vi "Leitura Weather160.vi"() -> (0 "Erro de Leitura=True":bool, 2 "Array":string[](array[string]))   [LabVIEW 2018]
uses:
  Global_Telescopio.vi
  <vilib>/Utility/error.llb/whitespace.ctl
  Shared_160.lvlib
panel:
  out "sizeFile":i32
  out "sizeCte":i32
  out "error out":errorcluster
  out "Ultima linha":string
  out "Saida":string
  # "Temp     Hi      Low     Out    Dew  Wind  Wind   Wind    Hi    Hi   Wind   Heat  THW  THSW             Solar   Solar   Hi Solar   UV    UV      Hi     Heat    Cool    In           In          In       In    Wind  Wind   ISS   Arc.\n  Date    Time     Out   Temp   Temp   Hum    Pt.  Speed   Dir      Run  Speed   Dir  Chill  Index  Index  Index    Bar     Rad.  Energy    Rad.  Index  Dose   UV     D-D     D-D    Temp   Hum    Dew   Heat     ET   Samp   Tx   Recept  Int."
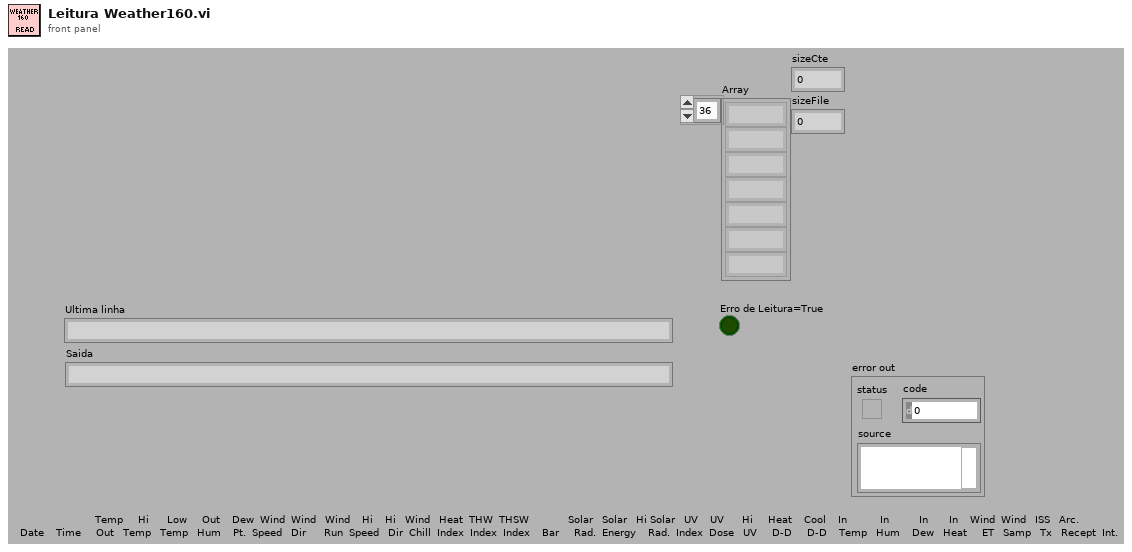
[diagram p1: front panel]
types:
  T1 = enum16{"open", "open or create", "create or replace", "create"}
  T2 = cluster{"broker":string, "version":string, "date":string, "hour":string, "outTemp":string, "hiTemp":string, "lowTemp":string, "outHumidity":string, "dewOut":string, "windSpeed":string, "windDirection":string, "windRun":string, "hiSpeed":string, "hiDir":string, "windChill":string, "heatIndex":string, "THWIndex":string, "THSIndex":string, "pressure":string, "rain":string, "rainRate":string, "solarRad":string, "solarEnergy":string, "hiSolarRad":string, "UVIndex":string, "UVDose":string, "hiUV":string, "headDD":string, "coolDD":string, "inTemp":string, "inHumidity":string, "inHeat":string, "inEMC":string, "inAirDensity":string, "2ndTemp":string, "2ndHumidity":string, "ET":string, "leaf":string, "windSamp":string, "windTx":string, "ISSRecept":string, "dewIn":string, "arcInt":string}
  T3 = typedef "whitespace.ctl" = u16
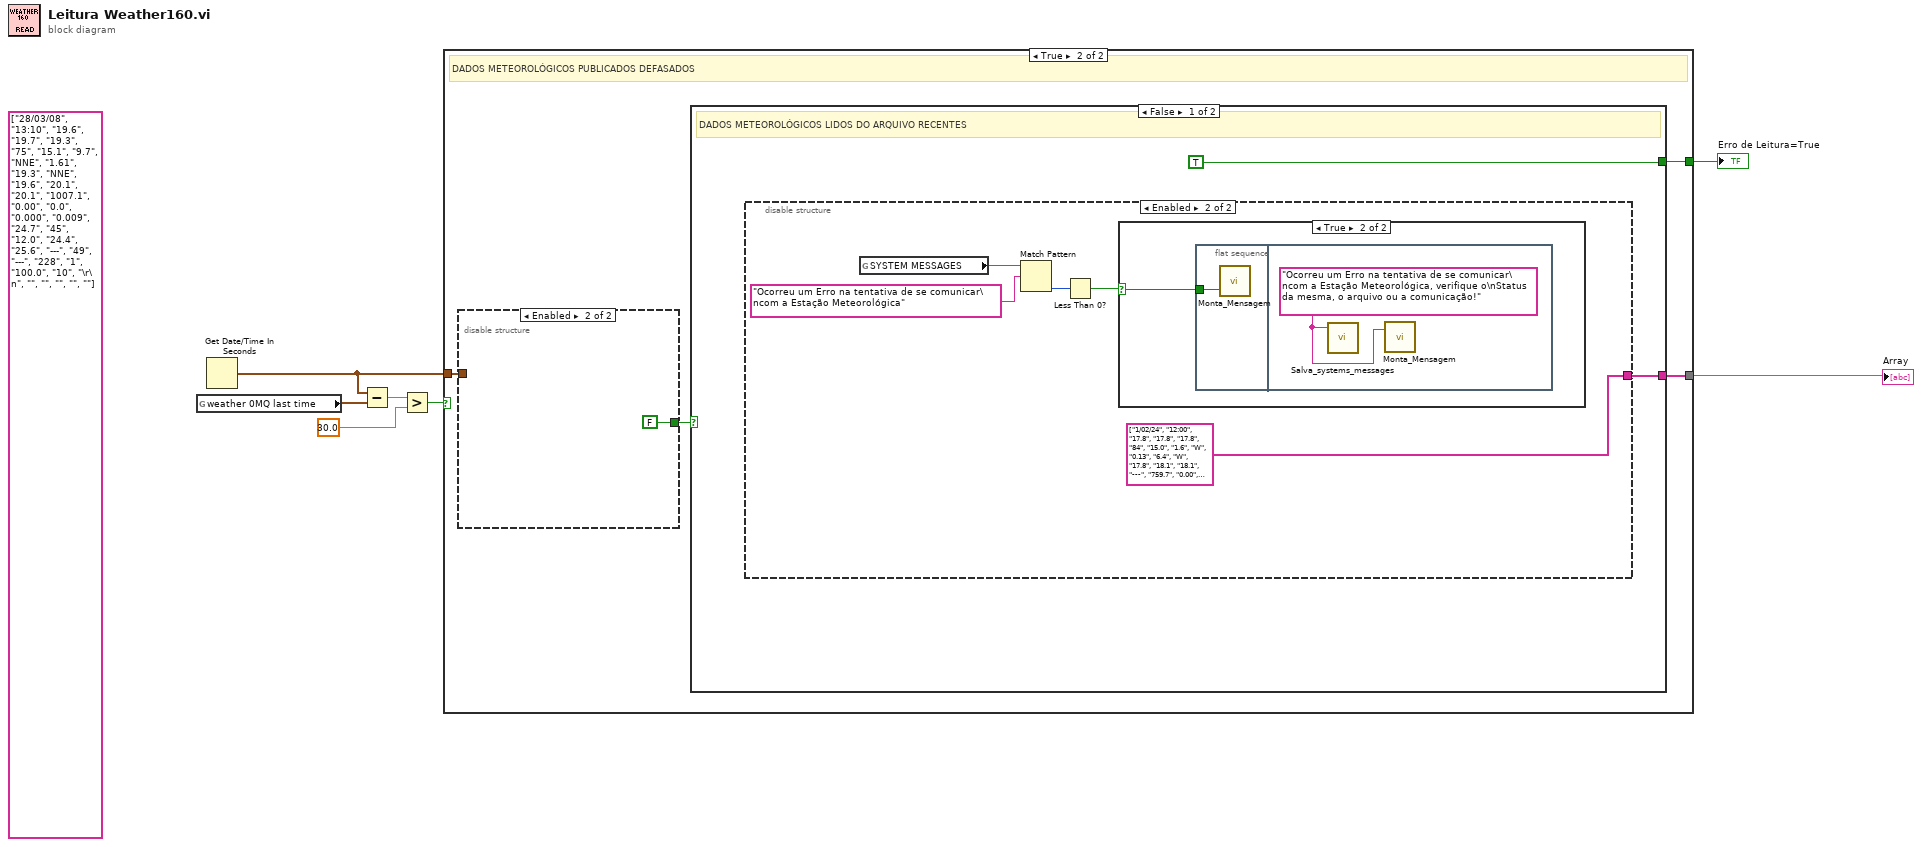
[diagram p0: block diagram]
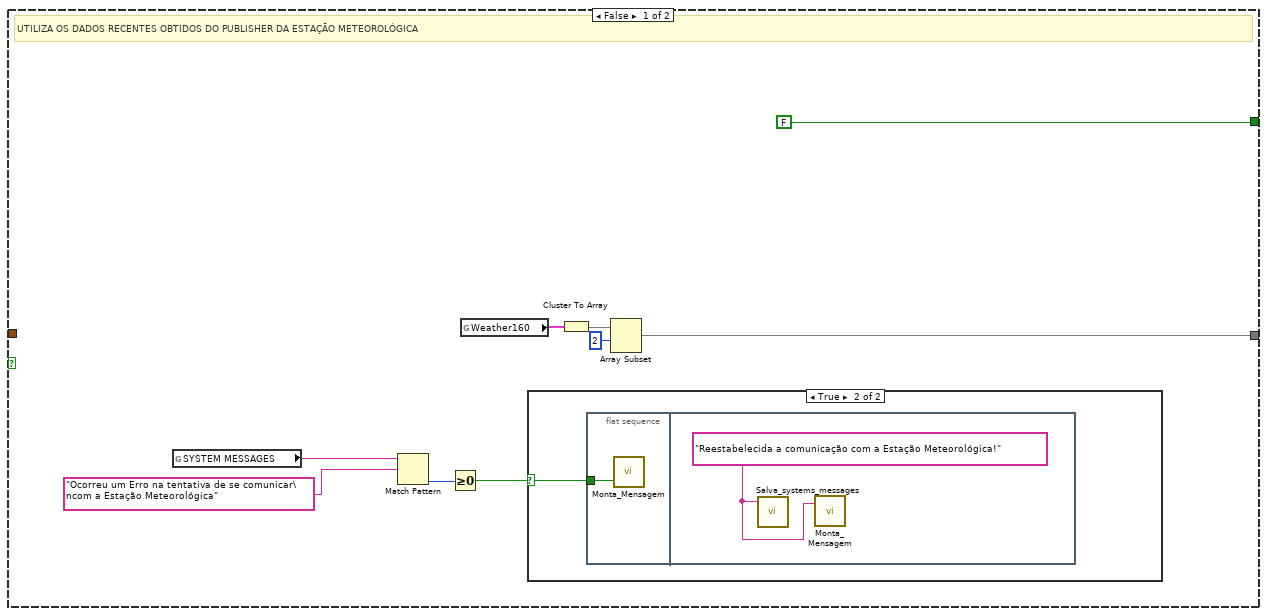
[diagram p2: hidden frame]
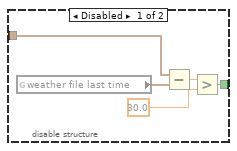
[diagram p4: hidden frame]
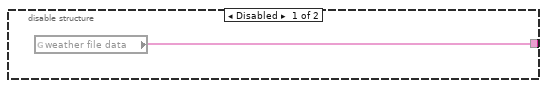
[diagram p5: hidden frame]
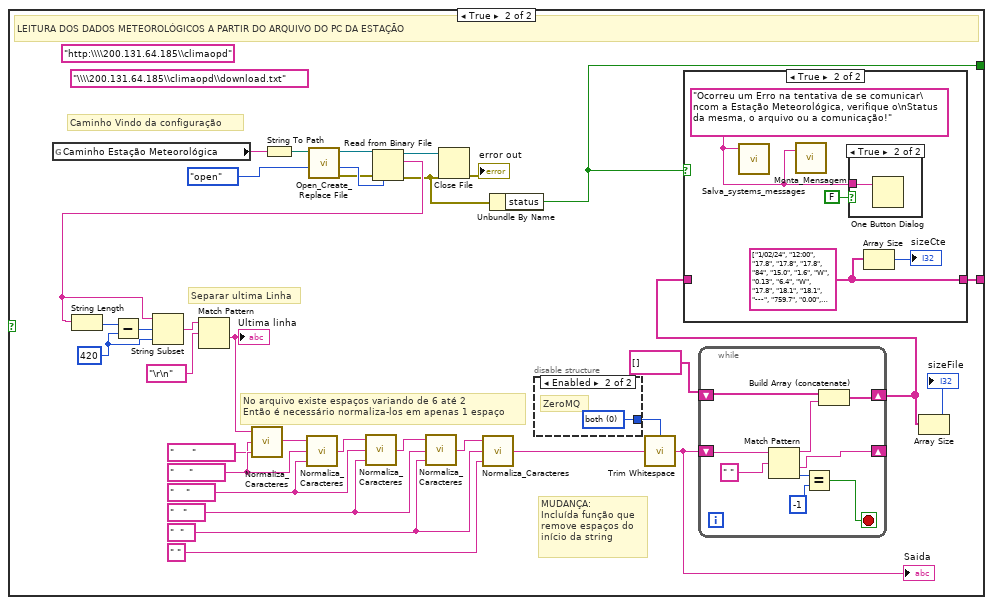
[diagram p7: hidden frame]
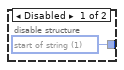
[diagram p8: hidden frame]
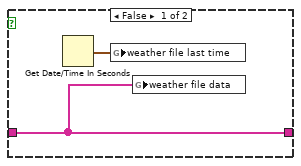
[diagram p9: hidden frame]
diagram:
  (unwired) string[] ["28/03/08", "13:10", "19.6", "19.7", "19.3", "75", "15.1", "9.7", "NNE", "1.61", "19.3", "NNE", "19.6", "20.1", "20.1", "1007.1", "0.00", "0.0", "0.000", "0.009", "24.7", "45", "12.0", "24.4", "25.6", "---", "49", "---", "228", "1", "100.0", "10", "\r\n", "", "", "", "", ""] ("Array 2")
  n1 = global read "Global_Telescopio.vi" "weather 0MQ last time"() -> (w6:timestamp)
  n2 = Get Date/Time In Seconds() -> (seconds since 1Jan1904=w3:timestamp)
  n3 = Subtract(x=w3, y=w6) -> (x-y=w5:dbl)
  n4 = Greater?(x=w5, y=30.0) -> (0:w1:bool)
  n5 = case shown="True" w1 {
    tunnel: [w13 w23] -> w7
    tunnel: w3 -> [_ w22]
    tunnel: [FALSE w20] -> w2
    frame False {
      # "UTILIZA OS DADOS RECENTES OBTIDOS DO PUBLISHER DA ESTAÇÃO METEOROLÓGICA"
      n6 = global read "Global_Telescopio.vi" "SYSTEM MESSAGES"() -> (w11:string)
      n7 = Match Pattern(string=w11, regular expression="Ocorreu um Erro na tentativa de se comunicar\ncom a Estação Meteorológica" ("message")) -> (offset past match=w12:i32)  [unwired: 1 in, 3 out]
      n8 = Greater Or Equal To 0?(x=w12) -> (x >= 0?=w9:bool)
      n9 = global read "Global_Telescopio.vi" "Weather160"() -> (w16:T2)
      n10 = case shown="True" w9 {
        selector: w9 -> [_ w17]
        frame False {
        }
        frame True {
          n11 = flat-sequence {
            tunnel: w17 -> [w18]
            frame #0 {
              n12 = call "Monta_Mensagem.vi"("Zerar"=w18) -> ()  [unwired: 2 in]
            }
            frame #1 {
              w19 = "Reestabelecida a comunicação com a Estação Meteorológica!" ("message")
              n13 = call "Salva_systems_messages.vi"("Mensagem"=w19) -> ()  [unwired: 5 in]
              n14 = call "Monta_Mensagem.vi"("Mensagem"=w19) -> ()  [unwired: 2 in]
            }
          }
        }
      }
      n15 = Cluster To Array(cluster=w16) -> (array=w15:string[])
      n16 = Array Subset(array=w15, index=2) -> (w13:string[])  [unwired: 1 in]
    }
    frame True {
      # "DADOS METEOROLÓGICOS PUBLICADOS DEFASADOS"
      n17 = disable-structure shown="Enabled" {
        disable-tunnel: w22 -> [w27 _]
        disable-tunnel: [w24 FALSE] -> w21
        frame Disabled {
          n18 = global read "Global_Telescopio.vi" "weather file last time"() -> (w26:timestamp)
          n19 = Subtract(x=w27, y=w26) -> (x-y=w28:dbl)
          n20 = Greater?(x=w28, y=30.0) -> (0:w24:bool)
        }
        frame Enabled {
        }
      }
      n21 = case shown="False" w21 {
        tunnel: [w31 w47] -> w23
        tunnel: [TRUE w42] -> w20
        frame False {
          # "DADOS METEOROLÓGICOS LIDOS DO ARQUIVO RECENTES"
          n22 = disable-structure shown="Enabled" {
            disable-tunnel: [w32 string[] ["1/02/24", "12:00", "17.8", "17.8", "17.8", "84", "15.0", "1.6", "W", "0.13", "6.4", "W", "17.8", "18.1", "18.1", "---", "759.7", "0.00", "0.0", "302", "2.16", "364", "3.2", "0.11", "3.6", "0.002", "0.000", "22.6", "64", "15.5", "22.8", "11.65", "1.1730", "21.7", "58", "0.15", "0", "114", "1", "100.0", "5"] ("Array 2")] -> w31
            frame Disabled {
              n23 = global read "Global_Telescopio.vi" "weather file data"() -> (w32:string[])
            }
            frame Enabled {
              n24 = global read "Global_Telescopio.vi" "SYSTEM MESSAGES"() -> (w36:string)
              n25 = Match Pattern(string=w36, regular expression="Ocorreu um Erro na tentativa de se comunicar\ncom a Estação Meteorológica" ("message")) -> (offset past match=w33:i32)  [unwired: 1 in, 3 out]
              n26 = Less Than 0?(x=w33) -> (x < 0?=w34:bool)
              n27 = case shown="True" w34 {
                selector: w34 -> [_ w38]
                frame False {
                }
                frame True {
                  n28 = flat-sequence {
                    tunnel: w38 -> [w39]
                    frame #0 {
                      n29 = call "Monta_Mensagem.vi"("Zerar"=w39) -> ()  [unwired: 2 in]
                    }
                    frame #1 {
                      w40 = "Ocorreu um Erro na tentativa de se comunicar\ncom a Estação Meteorológica, verifique o\nStatus da mesma, o arquivo ou a comunicação!" ("message")
                      n30 = call "Salva_systems_messages.vi"("Mensagem"=w40) -> ()  [unwired: 5 in]
                      n31 = call "Monta_Mensagem.vi"("Mensagem"=w40) -> ()  [unwired: 2 in]
                    }
                  }
                }
              }
            }
          }
        }
        frame True {
          w56 = 420 ("y")
          (unwired) "http:\\\\200.131.64.185\\climaopd"
          (unwired) "\\\\200.131.64.185\\climaopd\\download.txt" ("caminho final")
          w63 = "     "
          w67 = "  "
          w64 = "    "
          w68 = "   "
          # "MUDANÇA:\nIncluída função que\nremove espaços do\ninício da string"
          # "Caminho Vindo da configuração"
          # "Separar ultima Linha"
          # "No arquivo existe espaços variando de 6 até 2\nEntão é necessário normaliza-los em apenas 1 espaço"
          # "LEITURA DOS DADOS METEOROLÓGICOS A PARTIR DO ARQUIVO DO PC DA ESTAÇÃO"
          n32 = global read "Global_Telescopio.vi" "Caminho Estação Meteorológica"() -> (w51:string)
          n33 = String To Path(string=w51) -> (path=w59:path)
          n34 = call <vilib>:"Open_Create_Replace File.vi"("function (open:0)"=T1."open", "file path"=w59) -> ("error out"=w50:errorcluster, "file size (bytes)"=w73:i32, "refnum"=w71:refnum<file>)  [unwired: 6 in, 1 out]
          n35 = Read from Binary File(8:w50, 10:w73, 11:w71) -> (0:w41:errorcluster, 2:w55:string, 3:w72:refnum<file>)  [unwired: 3 in, 1 out]
          n36 = String Length(string=w55) -> (length=w58:i32)
          n37 = Subtract(x=w58, y=w56) -> (x-y=w57:i32)
          n38 = String Subset(string=w55, offset (0)=w57, length (rest)=w56) -> (substring=w54:string)
          n39 = Match Pattern(string=w54, regular expression="\r\n") -> (after substring=w52:string)  [unwired: 1 in, 3 out]
          "Ultima linha" <- w52
          n40 = call "Normaliza_Caracteres.vi"("Trocar por:"=w63, "Procurar"="      ", "Entrada"=w52) -> ("Saida"=w61:string)  [unwired: 2 in]
          n41 = call "Normaliza_Caracteres.vi"("Trocar por:"=w64, "Procurar"=w63, "Entrada"=w61) -> ("Saida"=w65:string)  [unwired: 2 in]
          n42 = call "Normaliza_Caracteres.vi"("Trocar por:"=w68, "Procurar"=w64, "Entrada"=w65) -> ("Saida"=w70:string)  [unwired: 2 in]
          n43 = call "Normaliza_Caracteres.vi"("Trocar por:"=w67, "Procurar"=w68, "Entrada"=w70) -> ("Saida"=w69:string)  [unwired: 2 in]
          n44 = Close File(refnum=w72, error in=w41) -> (error out=→"error out":errorcluster)  [unwired: 1 out]
          n45 = call "Normaliza_Caracteres.vi"("Trocar por:"=" ", "Procurar"=w67, "Entrada"=w69) -> ("Saida"=w48:string)  [unwired: 2 in]
          n46 = Unbundle By Name(w41) -> ("status"=w42:bool)
          n47 = disable-structure shown="Enabled" {
            disable-tunnel: [w75 w76] -> w45
            frame Disabled {
              w75 = T3 1 items=["both", "start of string", "end of string"] ("location (both)")
            }
            frame Enabled {
              w76 = T3 0 items=["both", "start of string", "end of string"] ("location (both)")
              # "ZeroMQ"
            }
          }
          n48 = call <vilib>:"Trim Whitespace.vi"("string"=w48, "location (both)"=w45) -> ("trimmed string"=w49:string)
          "Saida" <- w49
          n49 = while {
            shift-right: [w86] -> _
            shift-left: w49 -> [w87]
            shift-right: [w85] -> w44
            shift-left: string[] [] -> [w84]
            stop <- w88 stop-if-true
            n50 = Match Pattern(string=w87, regular expression=" ") -> (before substring=w92:string, after substring=w86:string, offset past match=w90:i32)  [unwired: 1 in, 1 out]
            n51 = Equal?(x=w90, y=-1) -> (x = y?=w88:bool)
            n52 = Build Array (concatenate)(w84, w92) -> (w85:string[])
          }
          n53 = case shown="True" w42 {
            tunnel: w44 -> [w77 _]
            tunnel: [w77 w81] -> w47
            frame False {
              n54 = Get Date/Time In Seconds() -> (seconds since 1Jan1904=w78:timestamp)
              n55 = global write "Global_Telescopio.vi" "weather file last time"(w78) -> ()
              n56 = global write "Global_Telescopio.vi" "weather file data"(w77) -> ()
            }
            frame True {
              w81 = string[] ["1/02/24", "12:00", "17.8", "17.8", "17.8", "84", "15.0", "1.6", "W", "0.13", "6.4", "W", "17.8", "18.1", "18.1", "---", "759.7", "0.00", "0.0", "302", "2.16", "364", "3.2", "0.11", "3.6", "0.002", "0.000", "22.6", "64", "15.5", "22.8", "11.65", "1.1730", "21.7", "58", "0.15", "0", "114", "1", "100.0", "5"] ("Array 2")
              w82 = "Ocorreu um Erro na tentativa de se comunicar\ncom a Estação Meteorológica, verifique o\nStatus da mesma, o arquivo ou a comunicação!" ("message")
              n57 = call "Salva_systems_messages.vi"("Mensagem"=w82) -> ()  [unwired: 5 in]
              n58 = call "Monta_Mensagem.vi"("Mensagem"=w82) -> ()  [unwired: 2 in]
              n59 = case shown="True" FALSE {
                tunnel: w82 -> [_ w83]
                frame False {
                }
                frame True {
                  n60 = One Button Dialog(message=w83) -> ()  [unwired: 1 in, 1 out]
                }
              }
              n61 = Array Size(array=w81) -> (size(s)=→"sizeCte":i32)
            }
          }
          n62 = Array Size(array=w44) -> (size(s)=→"sizeFile":i32)
        }
      }
    }
  }
  "Array" <- w7
  "Erro de Leitura=True" <- w2
